vi "Test - cameraV1 - Cam Image Response 1.vi"(8 "error in":errorcluster, 11 "Module ID":i32) -> (0 "error out":errorcluster, 3 "Pass":bool)   [LabVIEW 2024]
doc: "_____\nCreated using DQMH Framework: Event Scripter 7.1.0.1503."
uses:
  Libraries/cameraV1/cameraV1.lvlib
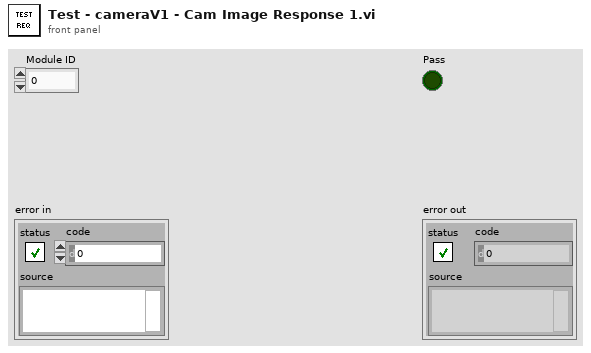
[diagram p1: front panel]
types:
  T1 = typedef "cameraV1.lvlib/Broadcast Events--cluster.ctl" = cluster{"Module Did Init":refnum<user-event>, "Status Updated":refnum<user-event>, "Error Reported":refnum<user-event>, "Module Did Stop":refnum<user-event>, "Update Module Execution Status":refnum<user-event>, "out reselt":refnum<user-event>}
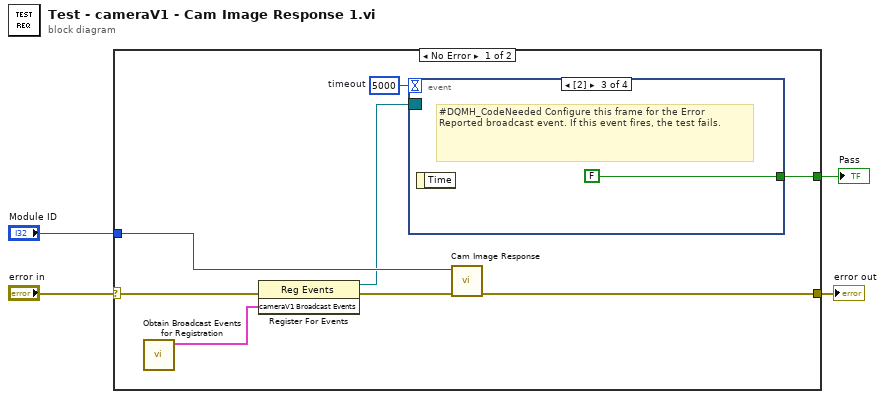
[diagram p0: block diagram]
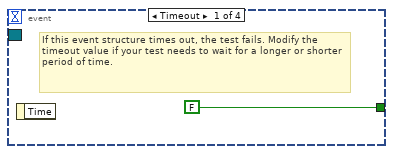
[diagram p2: hidden frame]
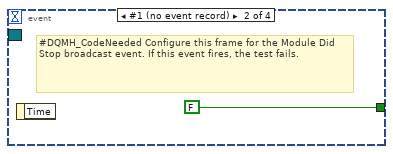
[diagram p3: hidden frame]
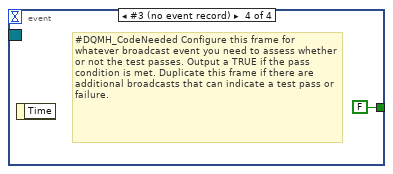
[diagram p4: hidden frame]
diagram:
  n1 = case shown="No Error" "error in" {
    selector: "error in" -> [w12 w17]
    tunnel: [w11 w17] -> w3
    tunnel: "Module ID" -> [w10 _]
    tunnel: [w5 _] -> w1
    frame No Error {
      w6 = 5000  # timeout
      n2 = call "Obtain Broadcast Events for Registration.vi"() -> ("cameraV1 Broadcast Events"=w8:T1)  [unwired: 9 in, 2 out]
      n3 = register-events(error in=w12, w8) -> (reference out=w7:refnum<event-registration>, error out=w9:errorcluster)  [unwired: 1 in]
      n4 = event shown="[2]" {
        selector: w7 -> [_ _ _ _]
        dyn-events: _ -> [_ _ _ _]
        timeout: w6 -> [_ _ _ _]
        tunnel: [FALSE FALSE FALSE FALSE] -> w5
        event Timeout {
          # "If this event structure times out, the test fails. Modify the timeout value if your test needs to wait for a longer or shorter period of time."
          n5 = event-data() -> ()  [unwired: 1 in, 1 out]
        }
        event #1 (no event record) {
          # "#DQMH_CodeNeeded Configure this frame for the Module Did Stop broadcast event. If this event fires, the test fails."
          n6 = event-data() -> ()  [unwired: 1 in, 1 out]
        }
        event #2 (no event record) {
          # "#DQMH_CodeNeeded Configure this frame for the Error Reported broadcast event. If this event fires, the test fails."
          n7 = event-data() -> ()  [unwired: 1 in, 1 out]
        }
        event #3 (no event record) {
          # "#DQMH_CodeNeeded Configure this frame for whatever broadcast event you need to assess whether or not the test passes. Output a TRUE if the pass condition is met. Duplicate this frame if there are additional broadcasts that can indicate a test pass or failure."
          n8 = event-data() -> ()  [unwired: 1 in, 1 out]
        }
      }
      n9 = call "Cam Image Response.vi"("error in"=w9, "Module ID"=w10) -> ("error out"=w11:errorcluster)  [unwired: 9 in]
    }
    frame Error {
    }
  }
  "error out" <- w3
  "Pass" <- w1
